vi "Scaled XOR Data.vi"() -> (4 "XOR":T1[](array[typedef]))   [LabVIEW 2011, in "Super Simple Neural Network.lvlib"]
uses:
  Super Simple Neural Network.lvlib
  Types/1D Array.ctl
  Types/Teaching Vector.ctl
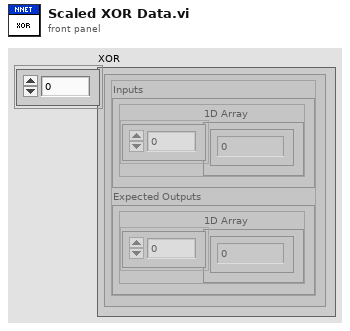
[diagram p1: front panel]
types:
  T1 = typedef "Super Simple Neural Network.lvlib/Teaching Vector.ctl" = cluster{"Inputs":T2, "Expected Outputs":T2}
  T2 = typedef "Super Simple Neural Network.lvlib/1D Array.ctl" = cluster{"1D Array":dbl[]}
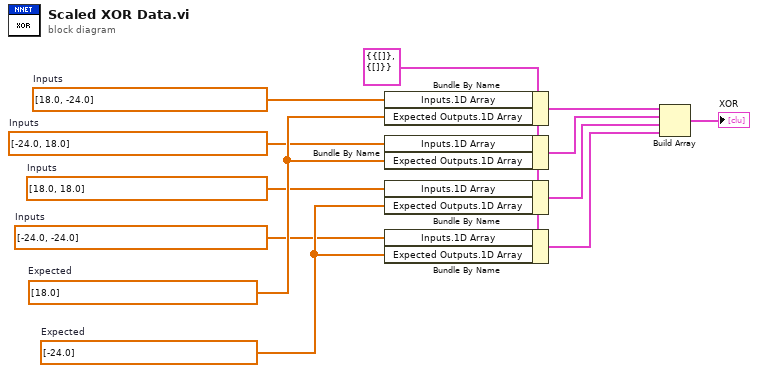
[diagram p0: block diagram]
diagram:
  w12 = T1 {"Inputs"={"1D Array"=[]}, "Expected Outputs"={"1D Array"=[]}}
  w11 = sgl[] [-24.0]  # Expected
  w5 = sgl[] [-24.0, -24.0]  # Inputs
  w4 = sgl[] [18.0, 18.0]  # Inputs
  w3 = sgl[] [-24.0, 18.0]  # Inputs
  w10 = sgl[] [18.0]  # Expected
  w2 = sgl[] [18.0, -24.0]  # Inputs
  n1 = Bundle By Name(cluster=w12, "Inputs.1D Array"=w2, "Expected Outputs.1D Array"=w10) -> (w6:T1)
  n2 = Bundle By Name(cluster=w12, "Inputs.1D Array"=w3, "Expected Outputs.1D Array"=w10) -> (w7:T1)
  n3 = Bundle By Name(cluster=w12, "Inputs.1D Array"=w4, "Expected Outputs.1D Array"=w11) -> (w8:T1)
  n4 = Bundle By Name(cluster=w12, "Inputs.1D Array"=w5, "Expected Outputs.1D Array"=w11) -> (w1:T1)
  n5 = Build Array(w6, w7, w8, w1) -> (→"XOR":T1[])
